vi "Caller.vi"(0 "Multiply in":refnum<class "Multiply.lvclass">, 2 "DVR In":refnum<data-value>, 5 "Sub Panel":refnum<vi>, 7 "State":refnum<user-event>, 9 "Class Data":refnum<user-event>, 11 "Error In":errorcluster) -> (4 "Multiply out":refnum<class "Multiply.lvclass">, 15 "Error Out":errorcluster)   [LabVIEW 2019, in "Multiply.lvclass"]
doc: "The VI asynchronously calls the Operation UI method of the multiplication operation."
uses:
  Multiply.lvclass
  Operation UI.vi
  Arithemtic Operation/Arithemetic Operation.lvclass
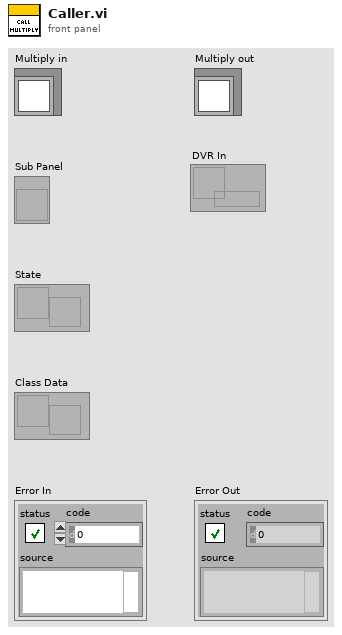
[diagram p1: front panel]
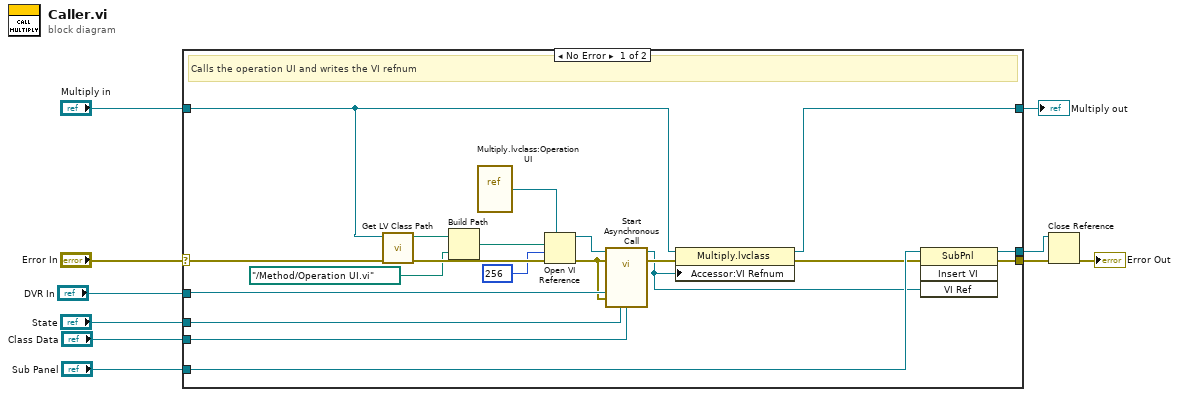
[diagram p0: block diagram]
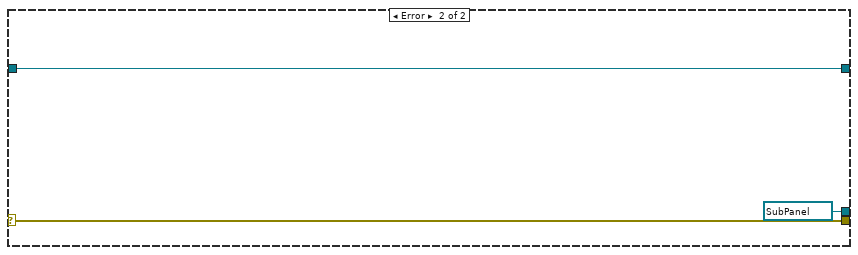
[diagram p2: hidden frame]
diagram:
  n1 = case shown="No Error" "Error In" {
    selector: "Error In" -> [w22 w33]
    tunnel: [w21 w33] -> w9
    tunnel: [w17 w32] -> w7
    tunnel: "Multiply in" -> [w15 w32]
    tunnel: "State" -> [w11 _]
    tunnel: "Class Data" -> [w12 _]
    tunnel: "Sub Panel" -> [w20 _]
    tunnel: [w16 refnum<vi> refnum ("Sub Panel")] -> w2
    tunnel: "DVR In" -> [w14 _]
    frame No Error {
      # "Calls the operation UI and writes the VI refnum"
      n2 = call <vilib>:"Get LV Class Path.vi"("error in (no error)"=w22, "object"=w15) -> ("error out"=w30:errorcluster, "class path"=w29:path)  [unwired: 8 in]
      n3 = Build Path(base path=w29, name or relative path=path "../Method/Operation UI.vi") -> (appended path=w27:path)
      n4 = vi-ref "Multiply.lvclass:Operation UI.vi"() -> (w23:refnum<vi>)
      n5 = Open VI Reference(type specifier VI Refnum (for type only)=w23, vi path=w27, options=256, error in (no error)=w30) -> (vi reference=w26:refnum<vi>, error out=w13:errorcluster)  [unwired: 2 in]
      n6 = call-by-ref "Start Asynchronous Call"(reference=w26, error in=w13, "DVR In"=w14, "Error In"=w13, "Stop"=w11, "Class Data"=w12) -> (reference out=w18:refnum<vi>, error out=w25:errorcluster)  [unwired: 9 in, 3 out]
      n7 = property class="Multiply.lvclass"(reference=w15, error in=w25, "Accessor:VI Refnum"=w18) -> (reference out=w17:refnum<class "Multiply.lvclass">, error out=w19:errorcluster)
      n8 = invoke on="Invoke Node" class="SubPnl" method="Insert VI"(reference=w20, error in=w19, "VI Ref"=w18) -> (reference out=w16:refnum<vi>, error out=w21:errorcluster)  [unwired: 1 in, 2 out]
    }
    frame Error {
    }
  }
  "Multiply out" <- w7
  n9 = Close Reference(reference=w2, error in (no error)=w9) -> (error out=→"Error Out":errorcluster)
